vi "Test_DataSetToVariantArraysDCluster.vi"() -> ()   [LabVIEW 2014, in "TableLogger_Actor.lvlib" / "TableLogger_Actor.lvclass"]
uses:
  TableLogger_Actor/TableLogger_Actor/TableLogger_Actor.lvclass
  TableLogger_SQLite_Actor.lvclass
panel:
  out "Label":string[](array[string])
  out "Value":string[](array[string])
  in  "LV Data":T1={"Numeric Data"=401, "Float Data"=0.0, "String Data"="", "Enum Data"=enum."Enum Item 1", "Array Data 2"=[0, 0, 0], "Cluster 2"={"String"="", "Array Data 2"=[0, 0, 0]}, "Cluster 3"={"Cluster78"={"Array Data 2"=[0, 0, 0]}}, "Enum Data 2"=enum."Enum Item 1", "String Data 2"="", "Float Data 2"=0.0, "Array Data"=[6, 0, 0, 4], "Array A"=[{"String A"="hello", "Array B"=[{"String B"="uq", "Array B 2"=[{"String B"="u"}, {"String B"="c"}, {"String B"="hello"}]}, {"String B"="c", "Array B 2"=[{"String B"="u"}, {"String B"="c"}, {"String B"="hello"}]}, {"String B"="hello", "Array B 2"=[{"String B"="u"}, {"String B"="c"}, {"String B"="hello"}]}], "Array B 2"=[{"String B"="u"}, {"String B"="c"}, {"String B"="hello"}]}, {"String A"="hello", "Array B"=[{"String B"="uP", "Array B 2"=[{"String B"="u"}, {"String B"="c"}, {"String B"="hello"}]}, {"String B"="c", "Array B 2"=[{"String B"="u"}, {"String B"="c"}, {"String B"="hello"}]}, {"String B"="hello", "Array B 2"=[{"String B"="u"}, {"String B"="c"}, {"String B"="hello"}]}], "Array B 2"=[{"String B"="u"}, {"String B"="c"}, {"String B"="hello"}]}]}
  out "Array":T2(array[cluster])
  out "Data":variant[](array[variant])
  in  "array":string[][](array[string])=[["Numeric Data", "Float Data", "String Data", "Enum Data", "Array Data 2[0].Numeric Data", "Array Data 2[1].Numeric Data", "Array Data 2[2].Numeric Data", "Cluster 2.String", "Cluster 2.Array Data 2[0].Numeric Data", "Cluster 2.Array Data 2[1].Numeric Data", "Cluster 2.Array Data 2[2].Numeric Data", "Cluster 3.Cluster78.Array Data 2[0].Numeric Data", "Cluster 3.Cluster78.Array Data 2[1].Numeric Data", "Cluster 3.Cluster78.Array Data 2[2].Numeric Data", "Enum Data 2", "String Data 2", "Float Data 2", "Array Data[0].Numeric Data", "Array Data[1].Numeric Data", "Array Data[2].Numeric Data", "Array Data[3].Numeric Data", "Array A[0].Cluster A.String A", "Array A[0].Cluster A.Array B[0].Cluster B.String B", "Array A[0].Cluster A.Array B[0].Cluster B.Array B 2[0].Cluster B.String B", "Array A[0].Cluster A.Array B[0].Cluster B.Array B 2[1].Cluster B.String B", "Array A[0].Cluster A.Array B[0].Cluster B.Array B 2[2].Cluster B.String B", "Array A[0].Cluster A.Array B[1].Cluster B.String B", "Array A[0].Cluster A.Array B[1].Cluster B.Array B 2[0].Cluster B.String B", "Array A[0].Cluster A.Array B[1].Cluster B.Array B 2[1].Cluster B.String B", "Array A[0].Cluster A.Array B[1].Cluster B.Array B 2[2].Cluster B.String B", "Array A[0].Cluster A.Array B[2].Cluster B.String B", "Array A[0].Cluster A.Array B[2].Cluster B.Array B 2[0].Cluster B.String B", "Array A[0].Cluster A.Array B[2].Cluster B.Array B 2[1].Cluster B.String B", "Array A[0].Cluster A.Array B[2].Cluster B.Array B 2[2].Cluster B.String B", "Array A[0].Cluster A.Array B 2[0].Cluster B.String B", "Array A[0].Cluster A.Array B 2[1].Cluster B.String B", "Array A[0].Cluster A.Array B 2[2].Cluster B.String B", "Array A[1].Cluster A.String A", "Array A[1].Cluster A.Array B[0].Cluster B.String B", "Array A[1].Cluster A.Array B[0].Cluster B.Array B 2[0].Cluster B.String B", "Array A[1].Cluster A.Array B[0].Cluster B.Array B 2[1].Cluster B.String B", "Array A[1].Cluster A.Array B[0].Cluster B.Array B 2[2].Cluster B.String B", "Array A[1].Cluster A.Array B[1].Cluster B.String B", "Array A[1].Cluster A.Array B[1].Cluster B.Array B 2[0].Cluster B.String B", "Array A[1].Cluster A.Array B[1].Cluster B.Array B 2[1].Cluster B.String B", "Array A[1].Cluster A.Array B[1].Cluster B.Array B 2[2].Cluster B.String B", "Array A[1].Cluster A.Array B[2].Cluster B.String B", "Array A[1].Cluster A.Array B[2].Cluster B.Array B 2[0].Cluster B.String B", "Array A[1].Cluster A.Array B[2].Cluster B.Array B 2[1].Cluster B.String B", "Array A[1].Cluster A.Array B[2].Cluster B.Array B 2[2].Cluster B.String B", "Array A[1].Cluster A.Array B 2[0].Cluster B.String B", "Array A[1].Cluster A.Array B 2[1].Cluster B.String B", "Array A[1].Cluster A.Array B 2[2].Cluster B.String B"], ["0", "0.0", "", "Enum Item 1", "0", "0", "0", "", "0", "0", "0", "0", "0", "0", "Enum Item 1", "", "0.0", "0", "0", "0", "4", "hello", "uq", "u", "c", "hello", "c", "u", "c", "hello", "hello", "u", "c", "hello", "u", "c", "hello", "hello", "uP", "u", "c", "hello", "c", "u", "c", "hello", "hello", "u", "c", "hello", "u", "c", "hello"], ["401", "0.0", "q", "Enum Item 1", "0", "0", "0", "", "0", "0", "0", "0", "0", "0", "Enum Item 1", "", "0.0", "0", "0", "0", "4", "hello", "uq", "u", "c", "hello", "c", "u", "c", "hello", "hello", "u", "c", "hello", "u", "c", "hello", "hello", "uP", "u", "c", "hello", "c", "u", "c", "hello", "hello", "u", "c", "hello", "u", "c", "hello"], ["0", "0.0", "", "Enum Item 1", "0", "0", "0", "", "0", "0", "0", "0", "0", "0", "Enum Item 1", "", "0.0", "0", "0", "0", "4", "hello", "uq", "u", "c", "hello", "c", "u", "c", "hello", "hello", "u", "c", "hello", "u", "c", "hello", "hello", "uP", "u", "c", "hello", "c", "u", "c", "hello", "hello", "u", "c", "hello", "u", "c", "hello"], ["0", "0.0", "", "Enum Item 1", "0", "0", "0", "", "0", "0", "0", "0", "0", "0", "Enum Item 1", "", "0.0", "0", "0", "0", "4", "hello", "uq", "u", "c", "hello", "c", "u", "c", "hello", "hello", "u", "c", "hello", "u", "c", "hello", "hello", "uP", "u", "c", "hello", "c", "u", "c", "hello", "hello", "u", "c", "hello", "u", "c", "hello"], ["0", "0.0", "", "Enum Item 1", "0", "0", "0", "", "0", "0", "0", "0", "0", "0", "Enum Item 1", "", "0.0", "0", "0", "0", "4", "hello", "uq", "u", "c", "hello", "c", "u", "c", "hello", "hello", "u", "c", "hello", "u", "c", "hello", "hello", "uP", "u", "c", "hello", "c", "u", "c", "hello", "hello", "u", "c", "hello", "u", "c", "hello"], ["0", "0.0", "", "Enum Item 1", "0", "0", "0", "", "0", "0", "0", "0", "0", "0", "Enum Item 1", "", "0.0", "0", "0", "0", "4", "hello", "uq", "u", "c", "hello", "c", "u", "c", "hello", "hello", "u", "c", "hello", "u", "c", "hello", "hello", "uP", "u", "c", "hello", "c", "u", "c", "hello", "hello", "u", "c", "hello", "u", "c", "hello"], ["0", "0.0", "", "Enum Item 1", "0", "0", "0", "", "0", "0", "0", "0", "0", "0", "Enum Item 1", "", "0.0", "0", "0", "0", "4", "hello", "uq", "u", "c", "hello", "c", "u", "c", "hello", "hello", "u", "c", "hello", "u", "c", "hello", "hello", "uP", "u", "c", "hello", "c", "u", "c", "hello", "hello", "u", "c", "hello", "u", "c", "hello"], ["0", "0.0", "", "Enum Item 1", "0", "0", "0", "", "0", "0", "0", "0", "0", "0", "Enum Item 1", "", "0.0", "0", "0", "0", "4", "hello", "uq", "u", "c", "hello", "c", "u", "c", "hello", "hello", "u", "c", "hello", "u", "c", "hello", "hello", "uP", "u", "c", "hello", "c", "u", "c", "hello", "hello", "u", "c", "hello", "u", "c", "hello"], ["0", "0.0", "", "Enum Item 1", "0", "0", "0", "", "0", "0", "0", "0", "0", "0", "Enum Item 1", "", "0.0", "0", "0", "0", "4", "hello", "uq", "u", "c", "hello", "c", "u", "c", "hello", "hello", "u", "c", "hello", "u", "c", "hello", "hello", "uP", "u", "c", "hello", "c", "u", "c", "hello", "hello", "u", "c", "hello", "u", "c", "hello"], ["0", "0.0", "", "Enum Item 1", "0", "0", "0", "", "0", "0", "0", "0", "0", "0", "Enum Item 1", "", "0.0", "0", "0", "0", "4", "hello", "uq", "u", "c", "hello", "c", "u", "c", "hello", "hello", "u", "c", "hello", "u", "c", "hello", "hello", "uP", "u", "c", "hello", "c", "u", "c", "hello", "hello", "u", "c", "hello", "u", "c", "hello"], ["0", "0.0", "", "Enum Item 1", "0", "0", "0", "", "0", "0", "0", "0", "0", "0", "Enum Item 1", "", "0.0", "0", "0", "0", "4", "hello", "uq", "u", "c", "hello", "c", "u", "c", "hello", "hello", "u", "c", "hello", "u", "c", "hello", "hello", "uP", "u", "c", "hello", "c", "u", "c", "hello", "hello", "u", "c", "hello", "u", "c", "hello"], ["401", "0.0", "", "Enum Item 1", "0", "0", "0", "", "0", "0", "0", "0", "0", "0", "Enum Item 1", "", "0.0", "0", "0", "0", "4", "hello", "uq", "u", "c", "hello", "c", "u", "c", "hello", "hello", "u", "c", "hello", "u", "c", "hello", "hello", "uP", "u", "c", "hello", "c", "u", "c", "hello", "hello", "u", "c", "hello", "u", "c", "hello"]]
  # "Array A[1].Array Data B[1].Numeric Data"
  # "Array A[0].Cluster A.Array Data B[0].Numeric Data"
  # "Cluster 3.Cluster 3.Cluster78.Cluster78.Array Data 2[0].Numeric Data"
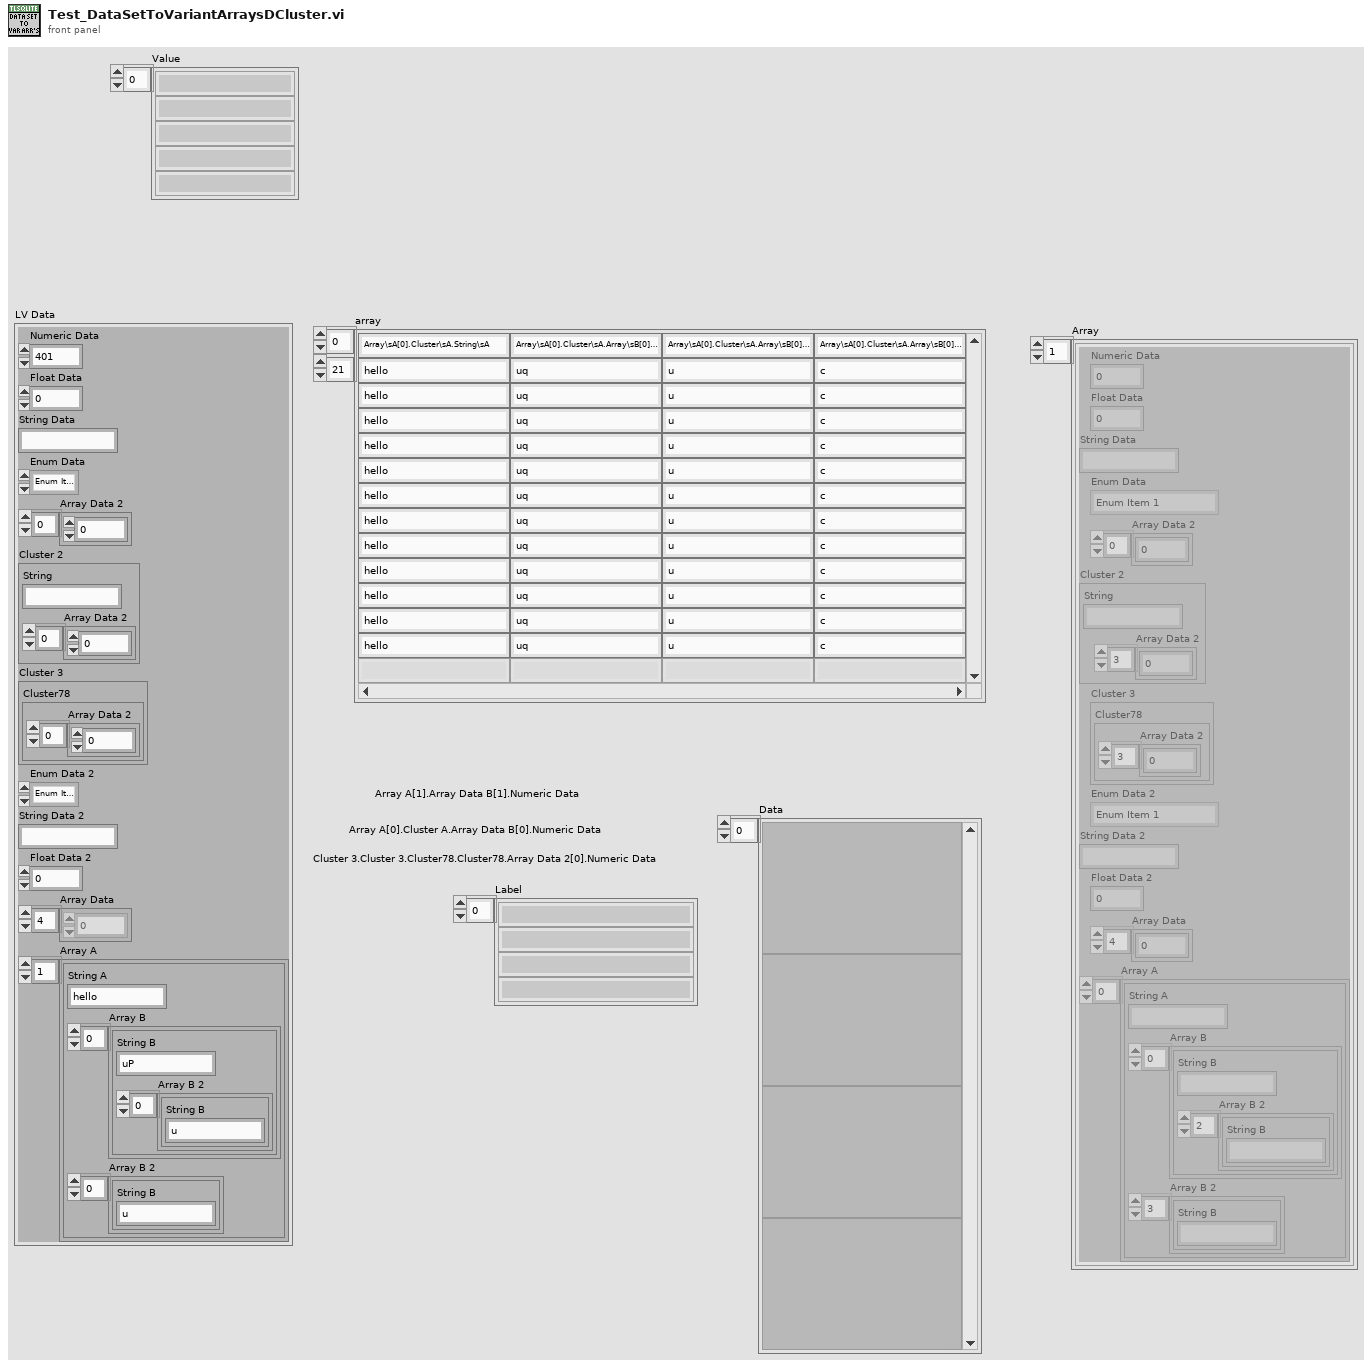
[diagram p1: front panel]
types:
  T1 = cluster{"Numeric Data":i32, "Float Data":dbl, "String Data":string, "Enum Data":enum16{"Enum Item 1", "Enum Item 2"}, "Array Data 2":i32[], "Cluster 2":cluster{"String":string, "Array Data 2":i32[]}, "Cluster 3":cluster{"Cluster78":cluster{"Array Data 2":i32[]}}, "Enum Data 2":enum16{"Enum Item 1", "Enum Item 2"}, "String Data 2":string, "Float Data 2":dbl, "Array Data":i32[], "Array A":cluster{"String A":string, "Array B":cluster{"String B":string, "Array B 2":cluster{"String B":string}[]}[], "Array B 2":cluster{"String B":string}[]}[]}
  T2 = cluster{"Numeric Data":i32, "Float Data":dbl, "String Data":string, "Enum Data":enum16{"Enum Item 1", "Enum Item 2"}, "Array Data 2":i32[], "Cluster 2":cluster{"String":string, "Array Data 2":i32[]}, "Cluster 3":cluster{"Cluster78":cluster{"Array Data 2":i32[]}}, "Enum Data 2":enum16{"Enum Item 1", "Enum Item 2"}, "String Data 2":string, "Float Data 2":dbl, "Array Data":i32[], "Array A":cluster{"String A":string, "Array B":cluster{"String B":string, "Array B 2":cluster{"String B":string}[]}[], "Array B 2":cluster{"String B":string}[]}[]}[]
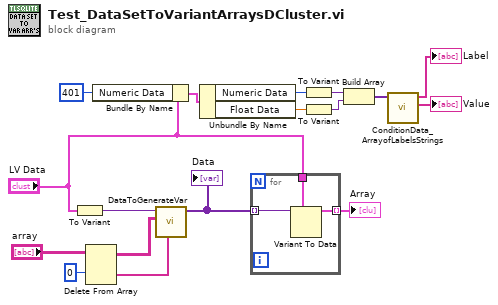
[diagram p0: block diagram]
diagram:
  n1 = To Variant(anything="LV Data") -> (Variant=w13:variant)
  n2 = Delete From Array(array="array", index (row)=0) -> (deleted portion=w14:string[], array with subset deleted=w16:string[][])  [unwired: 2 in]
  n3 = Bundle By Name(cluster="LV Data", "Numeric Data"=401) -> (w2:T1)
  n4 = call "DataToGenerateVar.vi"("Header"=w14, "Data in"=w16, "Variant"=w13) -> ("Data"=w17:variant[])  [unwired: 7 in, 1 out]
  "Data" <- w17
  n5 = Unbundle By Name(w2) -> ("Numeric Data"=w9:i32, "Float Data"=w8:dbl)
  n6 = for {
    tunnel: w17 -> [w20] mode=indexing
    tunnel: [w19] -> w11 mode=indexing
    tunnel: "LV Data" -> [w18]
    n7 = Variant To Data(type=w18, Variant=w20) -> (data=w19:T1)  [unwired: 1 in, 1 out]
  }
  "Array" <- w11
  n8 = To Variant(anything=w9) -> (Variant=w7:variant)
  n9 = To Variant(anything=w8) -> (Variant=w6:variant)
  n10 = Build Array(w7, w6) -> (w5:variant[])
  n11 = call "ConditionData_ArrayofLabelsStrings.vi"("Condition Data"=w5) -> ("Value"=→"Value":string[], "Label"=→"Label":string[])  [unwired: 8 in, 1 out]
